vi "Example.vi"() -> ()   [LabVIEW 2014]
uses:
  Private/Controls/Megger cluster.ctl
panel:
  in  "Abort":bool
  in  "Set time":i32=60
  in  "Set voltage":i32=4500
  out "Megger cluster":T1={"Read data"={"Firmware version"="", "Model number"="", "Serial number"=0, "Ramp rate"=0.0, "Test Voltage"=0.0, "Test duration"=0.0, "Test stop watch"=0.0, "measured Current (nA)"=0.0, "calculated Resistance"=0.0, "Test Mode"=enum."Insulation resistance (IR)", "Test status"=enum."Waiting to start test"}, "Connected?"=FALSE, "Device status array"=[]}
  in  "VISA resource name":refnum<visa-resource-name>
  in  "Close":bool
  in  "Start":bool
  # "User needs to select COM port before\nrunning the program. Or load from setup\nfile."
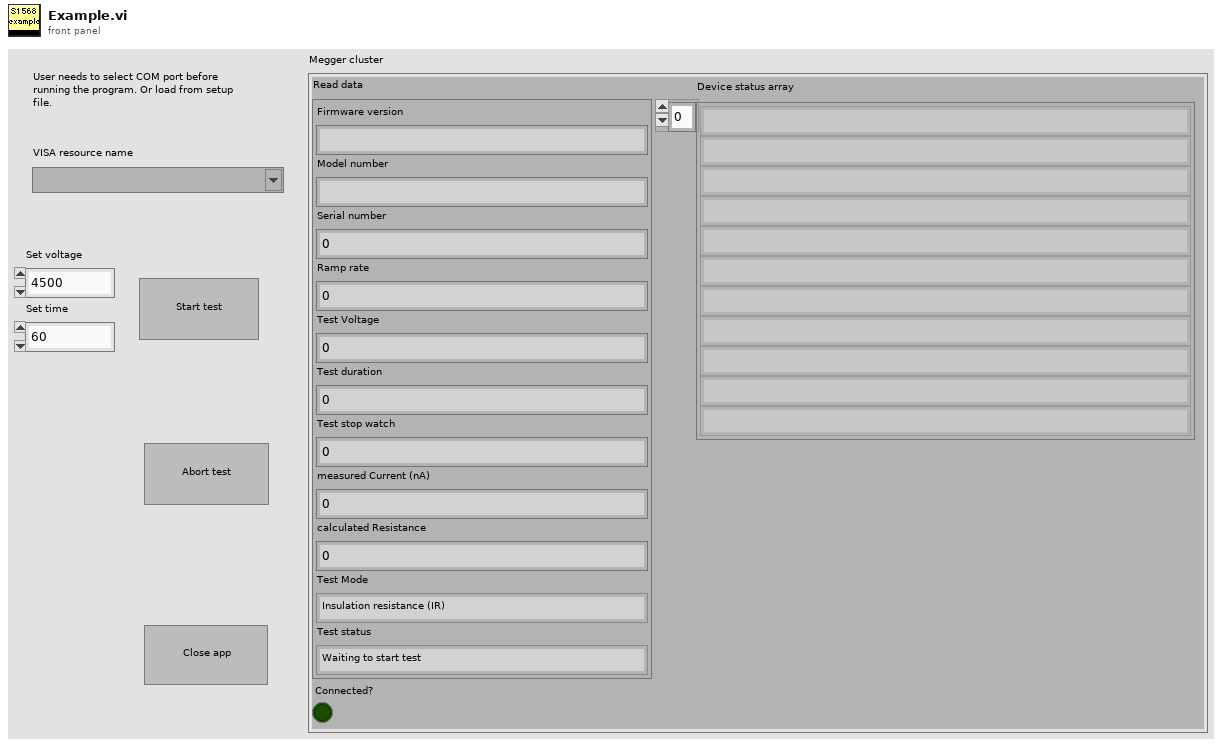
[diagram p1: front panel]
types:
  T1 = typedef "Megger cluster.ctl" = cluster{"Read data":cluster{"Firmware version":string, "Model number":string, "Serial number":i32, "Ramp rate":dbl, "Test Voltage":dbl, "Test duration":sgl, "Test stop watch":sgl, "measured Current (nA)":dbl, "calculated Resistance":dbl, "Test Mode":enum16{"N/A", "Insulation resistance (IR)", "Timed Insulation resistance (IR(t))", "Diaelectric Absorption Ratio (DAR)", "Polarisation Index (PI)", "Diaelectric Dishcharge (DD)", "Step voltage (SV)", "Ramp test (Ramp)"}, "Test status":enum16{"Waiting to start test", "Unable to start test", "Test progressing normally", "Performing post test measurements", "Test has ended normally", "Test has been aborted"}}, "Connected?":bool, "Device status array":string[]}
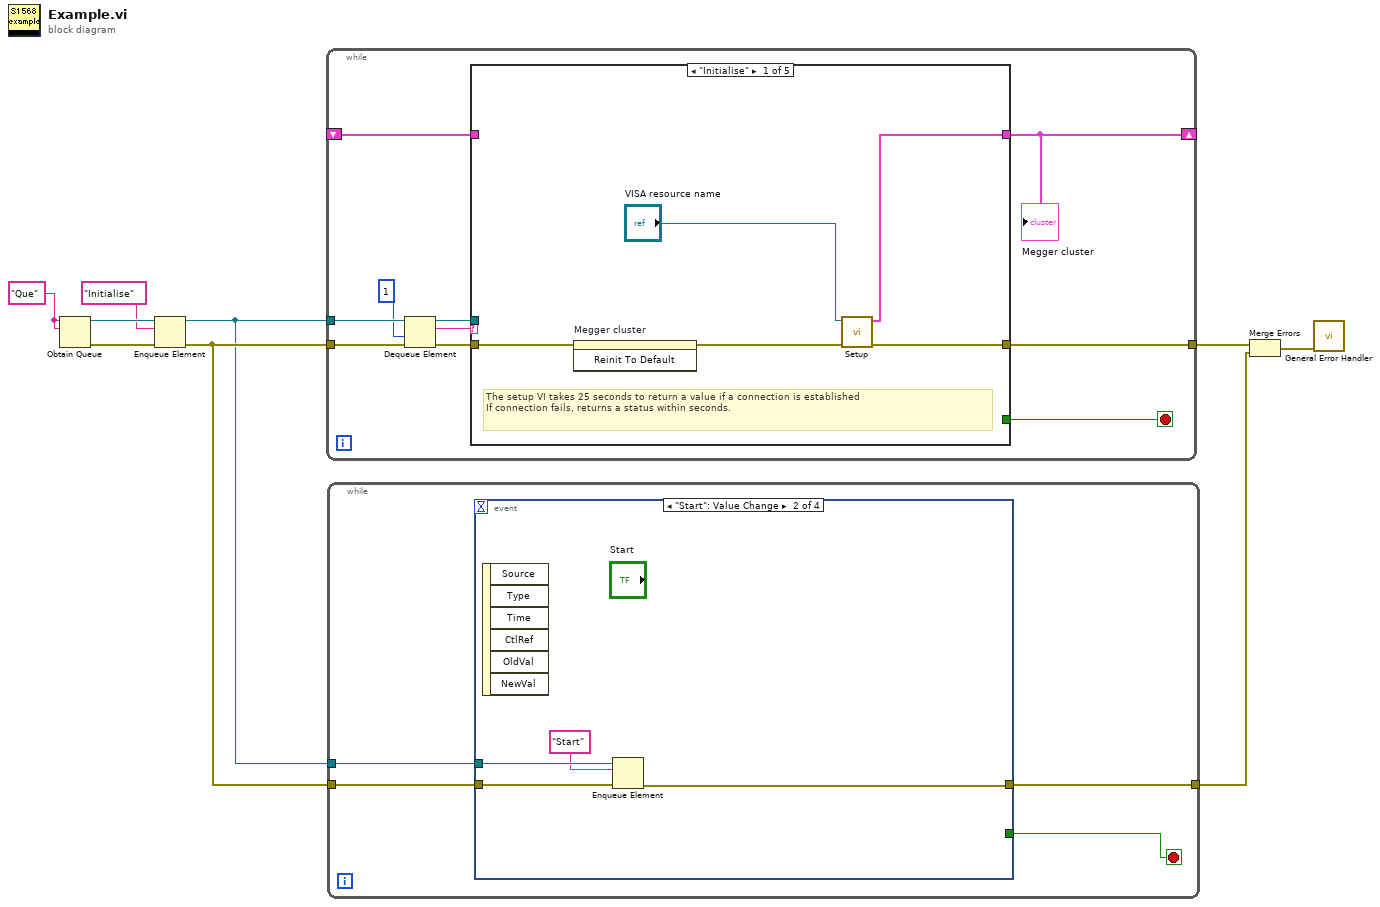
[diagram p0: block diagram]
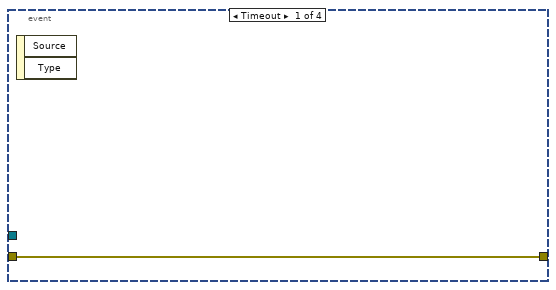
[diagram p2: hidden frame]
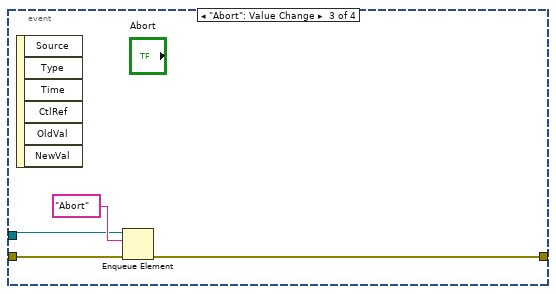
[diagram p3: hidden frame]
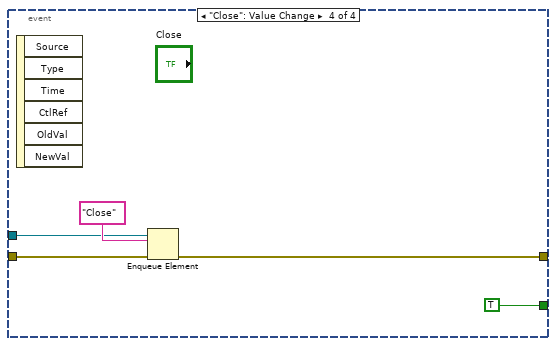
[diagram p4: hidden frame]
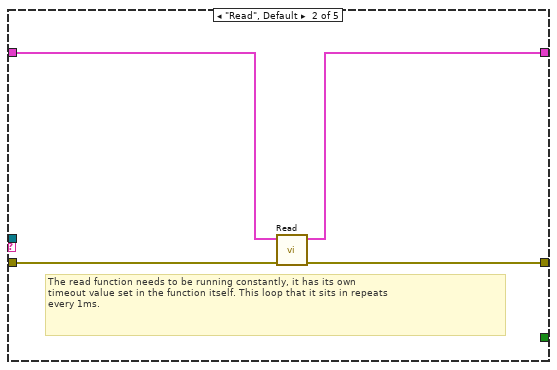
[diagram p5: hidden frame]
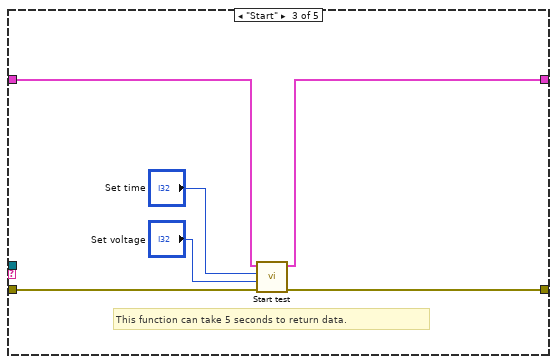
[diagram p6: hidden frame]
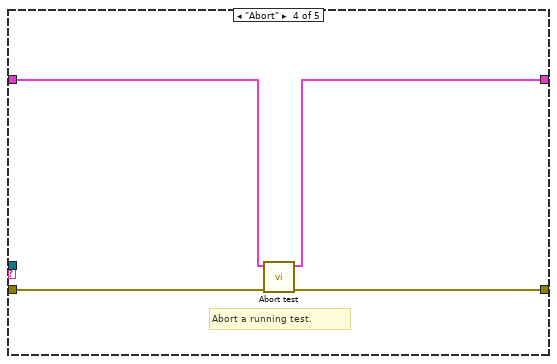
[diagram p7: hidden frame]
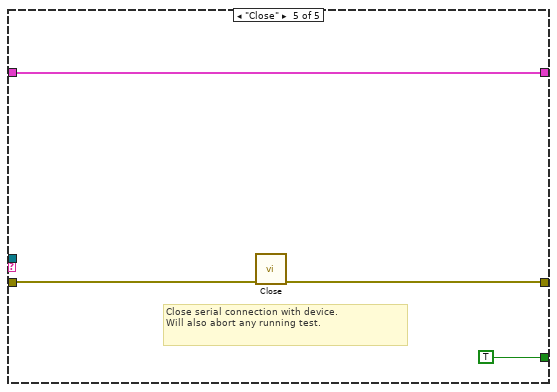
[diagram p8: hidden frame]
diagram:
  w9 = "Que" ("name (unnamed)")
  n1 = Obtain Queue(name (unnamed)=w9, element data type=w9) -> (queue out=w7:refnum<queue>, error out=w8:errorcluster)  [unwired: 3 in, 1 out]
  n2 = Enqueue Element(queue=w7, element="Initialise", error in (no error)=w8) -> (queue out=w1:refnum<queue>, error out=w2:errorcluster)  [unwired: 1 in, 1 out]
  n3 = while {
    tunnel: w2 -> [w17]
    tunnel: w1 -> [w19]
    tunnel: [w14] -> w5
    shift-right: [w11] -> _
    shift-left: _ -> [w10]
    stop <- w13 stop-if-true
    n4 = Dequeue Element(queue=w19, timeout in ms (-1)=1, error in (no error)=w17) -> (queue out=w18:refnum<queue>, element=w15:string, error out=w16:errorcluster)  [unwired: 1 out]
    n5 = case shown="\"Initialise\"" w15 {
      tunnel: w18 -> [_ _ _ _ _]
      tunnel: w16 -> [w21 w28 w34 w38 w40]
      tunnel: [w23 w27 w33 w37 w41] -> w14
      tunnel: [_ _ _ _ TRUE] -> w13
      tunnel: [w22 w25 w31 w35 w39] -> w11
      tunnel: w10 -> [_ w26 w32 w36 w39]
      frame "Initialise" {
        # "The setup VI takes 25 seconds to return a value if a connection is established\nIf connection fails, returns a status within seconds."
        n6 = invoke on="Megger cluster" class="Clust (strict)" method="Reinit To Default"(error in=w21) -> (error out=w20:errorcluster)  [unwired: 2 in, 2 out]
        n7 = call "Setup.vi"("error in"=w20, "VISA resource name"="VISA resource name") -> ("error out"=w23:errorcluster, "Megger cluster out"=w22:T1)  [unwired: 8 in]
      }
      frame "Read", Default {
        # "The read function needs to be running constantly, it has its own\ntimeout value set in the function itself. This loop that it sits in repeats\nevery 1ms."
        n8 = call "Read.vi"("error in"=w28, "Megger cluster in"=w26) -> ("error out"=w27:errorcluster, "Megger cluster out"=w25:T1)  [unwired: 8 in]
      }
      frame "Start" {
        # "This function can take 5 seconds to return data."
        n9 = call "Start test.vi"("error in"=w34, "Set voltage"="Set voltage", "Set time"="Set time", "Megger cluster in"=w32) -> ("error out"=w33:errorcluster, "Megger cluster out"=w31:T1)  [unwired: 6 in]
      }
      frame "Abort" {
        # "Abort a running test."
        n10 = call "Abort test.vi"("error in"=w38, "Megger cluster in"=w36) -> ("error out"=w37:errorcluster, "Megger cluster out"=w35:T1)  [unwired: 8 in]
      }
      frame "Close" {
        # "Close serial connection with device. \nWill also abort any running test."
        n11 = call "Close.vi"("error in"=w40) -> ("error out"=w41:errorcluster)  [unwired: 10 in]
      }
    }
    "Megger cluster" <- w11
  }
  n12 = while {
    tunnel: w2 -> [w46]
    tunnel: w1 -> [w45]
    tunnel: [w44] -> w4
    stop <- w43 stop-if-true
    n13 = event shown="[1] \"Start\": Value Change" {
      selector: _ -> [_ _ _ _]
      dyn-events: _ -> [_ _ _ _]
      timeout: _ -> [_ _ _ _]
      tunnel: w46 -> [w47 w51 w55 w59]
      tunnel: w45 -> [_ w50 w52 w57]
      tunnel: [w47 w48 w54 w58] -> w44
      tunnel: [_ _ _ TRUE] -> w43
      event Timeout {
        n14 = event-data() -> ()  [unwired: 1 in, 2 out]
      }
      event "Start": Value Change {
        n15 = event-data() -> ()  [unwired: 1 in, 6 out]
        n16 = Enqueue Element(queue=w50, element="Start", error in (no error)=w51) -> (error out=w48:errorcluster)  [unwired: 1 in, 2 out]
      }
      event "Abort": Value Change {
        n17 = event-data() -> ()  [unwired: 1 in, 6 out]
        n18 = Enqueue Element(queue=w52, element="Abort", error in (no error)=w55) -> (error out=w54:errorcluster)  [unwired: 1 in, 2 out]
      }
      event "Close": Value Change {
        n19 = event-data() -> ()  [unwired: 1 in, 6 out]
        n20 = Enqueue Element(queue=w57, element="Close", error in (no error)=w59) -> (error out=w58:errorcluster)  [unwired: 1 in, 2 out]
      }
    }
  }
  n21 = Merge Errors(w5, w4) -> (w3:errorcluster)
  n22 = call <vilib>:"General Error Handler.vi"("error in (no error)"=w3) -> ()  [unwired: 10 in, 5 out]
